vi "Motor State Machine.vi"(6 "Button D":bool, 7 "Button U":bool, 8 "Limit RD":bool, 9 "Limit RU":bool, 10 "Limit LD":bool, 11 "Limit LU":bool) -> (1 "Motor Out R":dbl, 2 "Motor Out L":dbl)   [LabVIEW 2014]
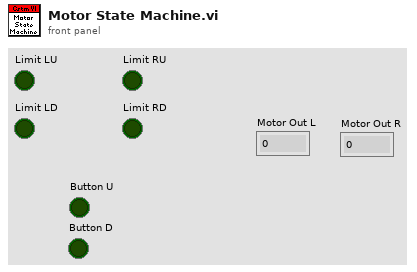
[diagram p1: front panel]
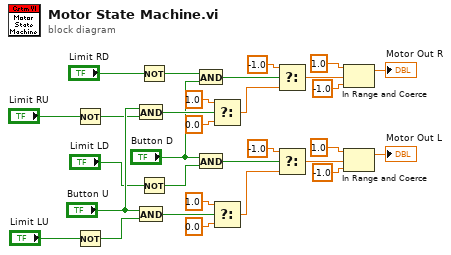
[diagram p0: block diagram]
diagram:
  n1 = Not(x="Limit RU") -> (.not. x?=w5:bool)
  n2 = Not(x="Limit LU") -> (.not. x?=w1:bool)
  n3 = And(x="Button U", y=w5) -> (x .and. y?=w14:bool)
  n4 = And(x="Button U", y=w1) -> (x .and. y?=w9:bool)
  n5 = Not(x="Limit RD") -> (.not. x?=w8:bool)
  n6 = Not(x="Limit LD") -> (.not. x?=w3:bool)
  n7 = And(x=w8, y="Button D") -> (x .and. y?=w13:bool)
  n8 = And(x="Button D", y=w3) -> (x .and. y?=w10:bool)
  n9 = Select(t=1.0, s=w14, f=0.0) -> (s? t:f=w19:dbl)
  n10 = Select(t=1.0, s=w9, f=0.0) -> (s? t:f=w26:dbl)
  n11 = Select(t=-1.0, s=w13, f=w19) -> (s? t:f=w20:dbl)
  n12 = Select(t=-1.0, s=w10, f=w26) -> (s? t:f=w27:dbl)
  n13 = In Range and Coerce(upper limit=1.0, x=w20, lower limit=-1.0) -> (coerced(x)=→"Motor Out R":dbl)  [unwired: 1 out]
  n14 = In Range and Coerce(upper limit=1.0, x=w27, lower limit=-1.0) -> (coerced(x)=→"Motor Out L":dbl)  [unwired: 1 out]
